vi "main_old.vi"() -> ()   [LabVIEW 2010]
panel:
  in  "LabVIEW._Application":refnum<k7>
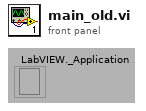
[diagram p1: front panel]
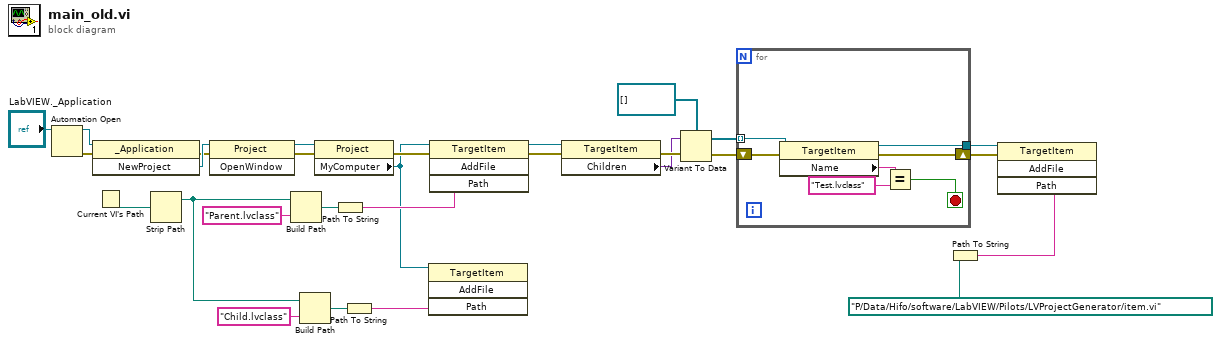
[diagram p0: block diagram]
diagram:
  n1 = Automation Open(Automation Refnum="LabVIEW._Application") -> (Automation Refnum=w25:refnum<k7>, error out=w24:errorcluster)  [unwired: 3 in]
  n2 = invoke on="Invoke Node" class="_Application" method="NewProject"(reference=w25, error in=w24) -> (error out=w26:errorcluster, "NewProject"=w27:refnum<k7>)  [unwired: 1 in, 1 out]
  n3 = Current VI's Path() -> (path=w9:path)
  n4 = Strip Path(path=w9) -> (stripped path=w3:path)  [unwired: 1 out]
  n5 = invoke on="Invoke Node" class="Project" method="OpenWindow"(reference=w27, error in=w26) -> (reference out=w22:refnum<k7>, error out=w23:errorcluster)  [unwired: 1 in, 1 out]
  n6 = Build Path(base path=w3, name or relative path="Parent.lvclass") -> (appended path=w8:path)
  n7 = Build Path(base path=w3, name or relative path="Child.lvclass") -> (appended path=w2:path)
  n8 = property class="Project"(reference=w22, error in=w23) -> (error out=w21:errorcluster, "MyComputer"=w5:refnum<k7>)  [unwired: 1 out]
  n9 = Path To String(path=w8) -> (string=w20:string)
  n10 = Path To String(path=w2) -> (string=w1:string)
  n11 = invoke on="Invoke Node" class="TargetItem" method="AddFile"(reference=w5, "Path"=w1) -> ()  [unwired: 2 in, 4 out]
  n12 = invoke on="Invoke Node" class="TargetItem" method="AddFile"(reference=w5, error in=w21, "Path"=w20) -> (reference out=w6:refnum<k7>, error out=w19:errorcluster)  [unwired: 1 in, 2 out]
  n13 = property class="TargetItem"(reference=w6, error in=w19) -> (error out=w18:errorcluster, "Children"=w16:variant)  [unwired: 1 out]
  n14 = Variant To Data(error in=w18, Variant=w16, type=refnum<k7>[] []) -> (error out=w15:errorcluster, data=w14:refnum<k7>[])
  n15 = for {
    shift-right: [w33] -> w12
    shift-left: w15 -> [w35]
    tunnel: w14 -> [w34] mode=indexing
    tunnel: [w29] -> w13
    stop <- w32 stop-if-true
    n16 = property class="TargetItem"(reference=w34, error in=w35) -> (reference out=w29:refnum<k7>, error out=w33:errorcluster, "Name"=w31:string)
    n17 = Equal?(x=w31, y="Test.lvclass") -> (x = y?=w32:bool)
  }
  n18 = Path To String(path=path "P:/Data/Hifo/software/LabVIEW/Pilots/LVProjectGenerator/item.vi") -> (string=w10:string)
  n19 = invoke on="Invoke Node" class="TargetItem" method="AddFile"(reference=w13, error in=w12, "Path"=w10) -> ()  [unwired: 1 in, 4 out]
